vi "Set Dynamic Parameters.vi"(8 "error in (no error)":errorcluster, 10 "dynamic parameters":cluster{"gear ratios":dbl[]}, 11 "Finger in":refnum<class "Finger.lvclass">) -> (0 "error out":errorcluster, 3 "Finger out":refnum<class "Finger.lvclass">)   [LabVIEW 2011, in "Finger.lvclass"]
uses:
  Finger.lvclass
  Finger.lvclass/Finger.ctl
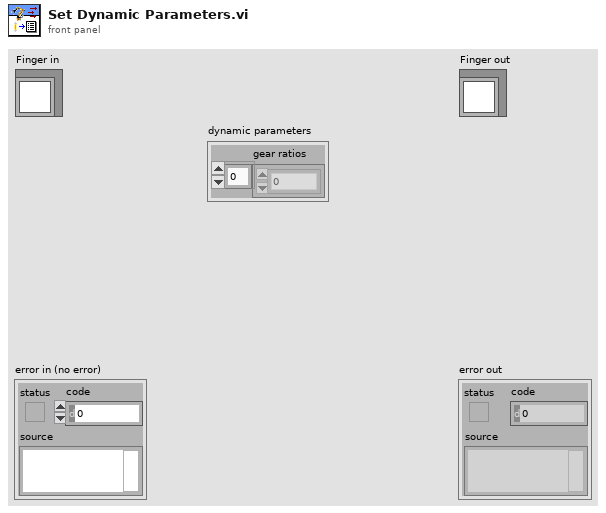
[diagram p1: front panel]
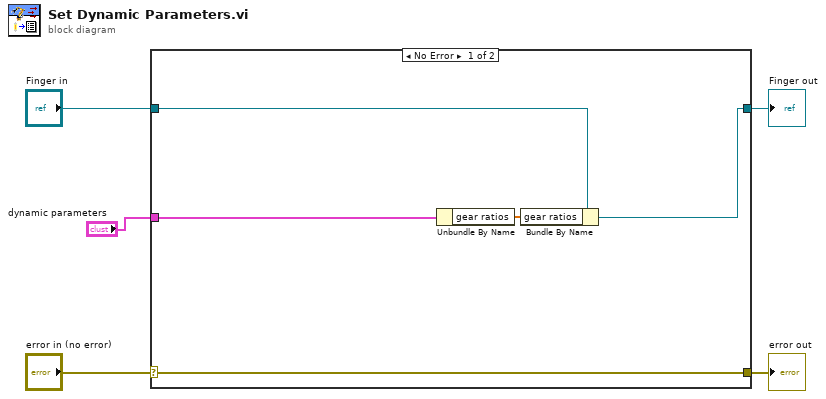
[diagram p0: block diagram]
diagram:
  n1 = case shown="No Error" "error in (no error)" {
    selector: "error in (no error)" -> [w10 w12]
    tunnel: [w10 w12] -> w4
    tunnel: [w6 w11] -> w2
    tunnel: "Finger in" -> [w9 w11]
    tunnel: "dynamic parameters" -> [w7 _]
    frame No Error {
      n2 = Unbundle By Name(w7) -> ("gear ratios"=w8:dbl[])
      n3 = Bundle By Name(cluster=w9, "gear ratios"=w8) -> (w6:refnum<class "Finger.lvclass">)
    }
    frame Error {
    }
  }
  "error out" <- w4
  "Finger out" <- w2
